vi "CommandFIFOMultiplexer.vi"   [LabVIEW 2018]
uses:
  <vilib>/rvi/Emulation/niFpgaGetClockAttributes.vi
  <vilib>/rvi/Emulation/niFpgaSctlEmulationGetInTimedLoop.vi
  <vilib>/rvi/Emulation/niFpgaEmulationReportErrorSimple.vi
  <vilib>/rvi/interface/RandomDataEmulation/niFpgaRandomDataHandleErrors.vi
  <vilib>/rvi/Emulation/niFpgaEmulationIsFPGAContextNoSignature.vi
  <vilib>/rvi/errors/niFpgaSetErrorForExecOnDevCompSimple.vi
  <vilib>/rvi/eio/common/nirviEmuReportErrorAndStop.vi
  <vilib>/rvi/DataTransferAndStorage/Container/Common/niFpgaContainerGetUniqueNameForEmu.vi
  <vilib>/rvi/FIFO/Fifo_Resource/nirvififoEmulationSetSize.vi
  <vilib>/rvi/FIFO/Fifo_Resource/nirviFifoEmulationQueueMgr.vi
  <instcachedir>/0/nirviFifoEmulationQueueMgr_E5CAEC123FF24DC58D834DCA3CDAA9B5.lvgen/nirviFifoEmulationQueueMgr_E5CAEC123FF24DC58D834DCA3CDAA9B5_001.vi
  <vilib>/rvi/FIFO/Fifo_Resource/nirvififoEmulationDetermineInputValidOut.vi
  <vilib>/rvi/FIFO/Fifo_Resource/nirvififoEmulationCreateLock.vi
  <vilib>/rvi/Emulation/niFpgaProcessEmulError.vi
  <vilib>/rvi/FIFO/Fifo_Resource/nirvififoEmulationObtainLock.vi
  <vilib>/rvi/FIFO/Fifo_Resource/nirvififoEmulationReleaseLock.vi
  <vilib>/rvi/occurrence/nirviWaitOnOccurrenceBase.vi
  <vilib>/rvi/errors/nirviReportUnexpectedCaseInternalError.vi
  <vilib>/rvi/errors/nirviReportUnexpectedCaseInternalError (U32).vi
  <vilib>/rvi/DataTransferAndStorage/Container/Common/niFpgaContainerExecOnDevCompGetState.vi
  <instcachedir>/0/nirviFifoEmulationQueueMgr_E5CAEC123FF24DC58D834DCA3CDAA9B5.lvgen/nirviFifoEmulationQueueMgr_E5CAEC123FF24DC58D834DCA3CDAA9B5_012.vi
  <vilib>/Utility/error.llb/Clear Errors.vi
  <vilib>/rvi/Emulation/niFpgaCriticalErrorInLSC.vi
  <vilib>/rvi/DataTransferAndStorage/Container/XNode/niFpgaContainer.xnode
  <vilib>/rvi/interface/RandomDataEmulation/nirviRandomDataFpgaReadWriteTemplate.vi
  <vilib>/rvi/FIFO/Fifo_Resource/nirvififoEmulationWrite.vi
  <vilib>/rvi/FIFO/Fifo_Resource/niFpgaFifoEmulationRefIn.vi
types:
  T1 = typedef "Addresses.ctl" = enum8{"NA", "Slot1/AI0-CT7Current", "Slot1/AI1-CT8Current", "Slot1/AI2", "Slot1/AI3", "Slot1/AI4", "Slot1/AI5", "Slot1/AI6", "Slot1/AI7", "Slot1/AI8-MixingValvePosition", "Slot1/AI9", "Slot1/AI10", "Slot1/AI11", "Slot1/AI12", "Slot1/AI13", "Slot1/AI14", "Slot1/AI15", "Slot2/AO0-MixingValvePosition", "Slot2/AO1", "Slot2/AO2", "Slot2/AO3", "Slot3/DIO0-ModbusARx", "Slot3/DIO1", "Slot3/DIO2", "Slot3/DIO3", "Slot3/DIO4-ModbusATx", "Slot3/DIO5", "Slot3/DIO6", "Slot3/DIO7", "Slot4/DI0-PS14Status", "Slot4/DI1-PS15Status", "Slot4/DI2-PS16Status", "Slot4/DI3-CtrlRedundancyStatus", "Slot4/DI4-FanCoilDiffuserStatus", "Slot4/DI5-ACPowerCB15Status", "Slot4/DI6-UtilityOutletCB18Status", "Slot4/DI7-CoolandPumpOLStatus", "Slot4/DI8", "Slot4/DI9", "Slot4/DI10", "Slot4/DI11", "Slot4/DI12", "Slot4/DI13", "Slot4/DI14", "Slot4/DI15", "Slot4/DI16-FCHeatersOffInterlock", "Slot4/DI17-CoolandPumpOffInterlock", "Slot4/DI18-GISHBLostInterlock", "Slot4/DI19-MixingValveClosedInterlock", "Slot4/DI20-SupportSystemHBLostInterlock", "Slot4/DI21-CellDoorOpenInterlock", "Slot4/DI22-GISEarthQuakeInterlock", "Slot4/DI23-CoolantPumpEStopInterlock", "Slot4/DI24-CabinetOverTempInterlock", "Slot4/DI25", "Slot4/DI26", "Slot4/DI27", "Slot4/DI28", "Slot4/DI29", "Slot4/DI30", "Slot4/DI31", "Slot5/Ch0-FanCoilHeatersOn", "Slot5/Ch1-ThermalHeartbeat", "Slot5/Ch2-CoolantPumpOn", "Slot5/Ch3", "Slot5/Ch4", "Slot5/Ch5", "Slot5/Ch6", "Slot5/Ch7", "Slot6/Port1-VFD", "Slot6/Port2-FlowMeter", "Slot6/Port3-WindSensor", "Slot6/Port4", "Slot7/Port1", "Slot7/Port2", "Slot7/Port3", "Slot7/Port4", "Slot8/TC0-AirMirrorTopSurface", "Slot8/TC1-MirrorCellAir", "Slot8/TC2-MirrorCoolantSupply", "Slot8/TC3-MirrorCoolandReturn", "Slot8/TC4-TelescopeCoolantSupply", "Slot8/TC5-TelescopeCoolantReturn", "Slot8/TC6", "Slot8/TC7", "Slot8/TC8", "Slot8/TC9", "Slot8/TC10", "Slot8/TC11", "Slot8/TC12", "Slot8/TC13", "Slot8/TC14", "Slot8/TC15", "Undefined17", "Undefined18", "Undefined19", "Undefined20", "Undefined21", "Undefined22", "Undefined23", "Undefined24", "Undefined25", "Undefined26", "Undefined27", "Undefined28", "Undefined29", "Undefined30", "Undefined31", "Undefined32", "Undefined33", "Undefined34", "Undefined35", "Undefined36", "Undefined37", "Undefined38", "Undefined39", "Undefined40", "Undefined41", "Undefined42", "Undefined43", "Undefined44", "Undefined45", "Undefined46", "Undefined47", "Undefined48", "Undefined49", "Undefined50", "Undefined51", "Undefined52", "Undefined53", "Undefined54", "Undefined55", "Undefined56", "Undefined57", "Undefined58", "Undefined59", "Undefined60", "Undefined61", "Undefined62", "Undefined63", "Undefined64", "Undefined65", "Undefined66", "Undefined67", "Undefined68", "Undefined69", "Undefined70", "Undefined71", "Undefined72", "Undefined73", "Undefined74", "Undefined75", "Undefined76", "Undefined77", "Undefined78", "Undefined79", "Undefined80", "Undefined81", "Undefined82", "Undefined83", "Undefined84", "Undefined85", "Undefined86", "Undefined87", "Undefined88", "Undefined89", "Undefined90", "Undefined91", "Undefined92", "Undefined93", "Undefined94", "Undefined95", "Undefined96", "Undefined97", "Undefined98", "Undefined99", "Undefined100", "Undefined101", "Undefined102", "Undefined103", "Undefined104", "Undefined105", "Undefined106", "Undefined107", "Undefined108", "Undefined109", "Undefined110", "Undefined111", "Undefined112", "Undefined113", "Undefined114", "Undefined115", "Undefined116", "Undefined117", "Undefined118", "Undefined119", "Undefined120", "Undefined121", "Undefined122", "Undefined123", "Undefined124", "Undefined125", "Undefined126", "Undefined127", "Undefined128", "Undefined129", "Undefined130", "Undefined131", "Undefined132", "Undefined133", "Undefined134", "Undefined135", "Undefined136", "Undefined137", "Undefined138", "Undefined139", "Undefined140", "Undefined141", "Undefined142", "Undefined143", "Undefined144", "Undefined145", "Undefined146", "Undefined147", "Undefined148", "Undefined149", "Undefined150", "Undefined151", "Undefined152", "Undefined153", "Undefined154", "Undefined155", "Undefined156", "Undefined157", "Undefined158", "Undefined159", "Undefined160", "Undefined161", "Undefined162", "Undefined163", "Undefined164", "Undefined165", "Undefined166", "Undefined167", "Undefined168", "Undefined169", "Undefined170", "Undefined171", "Undefined172", "Undefined173", "Undefined174", "Undefined175", "ModbusSoftwareTrigger", "Telemetry", "HealthAndStatus", "Timestamp"}
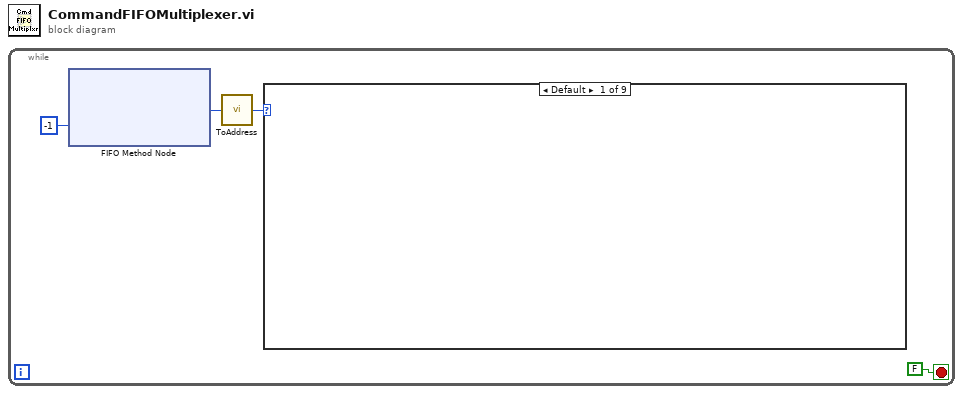
[diagram p0: block diagram]
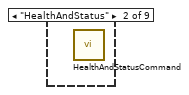
[diagram p2: hidden frame]
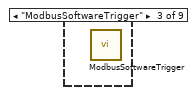
[diagram p3: hidden frame]
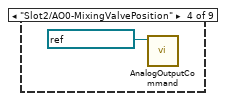
[diagram p4: hidden frame]
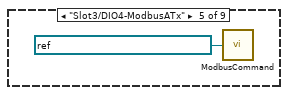
[diagram p5: hidden frame]
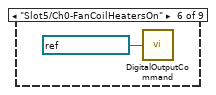
[diagram p6: hidden frame]
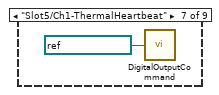
[diagram p7: hidden frame]
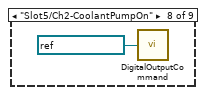
[diagram p8: hidden frame]
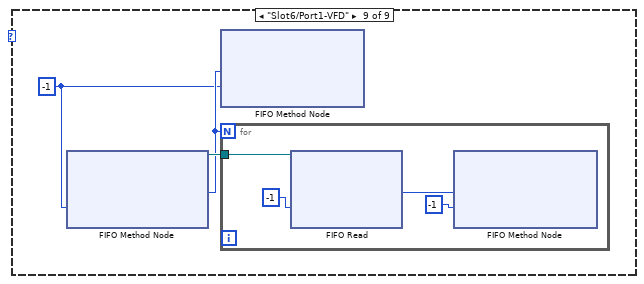
[diagram p9: hidden frame]
diagram:
  n1 = while {
    stop <- FALSE stop-if-true
    n2 = xnode ("FIFO Method Node")("Timeout"=-1) -> ("Element"=w3:u16)  [unwired: 1 in, 2 out]
    n3 = call "ToAddress.vi"("Input"=w3) -> ("Address"=w2:T1)
    n4 = case shown="Default" w2 {
      frame Default {
      }
      frame "HealthAndStatus" {
        n5 = call "HealthAndStatusCommand.vi"() -> ()  [unwired: 12 in]
      }
      frame "ModbusSoftwareTrigger" {
        n6 = call "ModbusSoftwareTrigger.vi"() -> ()  [unwired: 12 in]
      }
      frame "Slot2/AO0-MixingValvePosition" {
        n7 = call "AnalogOutputCommand.vi"("FPGA I/O In"=refnum<k21> "Mod2/AO0") -> ()  [unwired: 11 in]
      }
      frame "Slot3/DIO4-ModbusATx" {
        n8 = call "ModbusCommand.vi"("SubnetTxFIFO"=refnum<k21> "ModbusSubnetATxDataFIFO") -> ()  [unwired: 1 in]
      }
      frame "Slot5/Ch0-FanCoilHeatersOn" {
        n9 = call "DigitalOutputCommand.vi"("FPGA I/O In"=refnum<k21> "Mod5/CH0") -> ()  [unwired: 1 in]
      }
      frame "Slot5/Ch1-ThermalHeartbeat" {
        n10 = call "DigitalOutputCommand.vi"("FPGA I/O In"=refnum<k21> "Mod5/CH1") -> ()  [unwired: 1 in]
      }
      frame "Slot5/Ch2-CoolantPumpOn" {
        n11 = call "DigitalOutputCommand.vi"("FPGA I/O In"=refnum<k21> "Mod5/CH2") -> ()  [unwired: 1 in]
      }
      frame "Slot6/Port1-VFD" {
        w10 = -1 ("Timeout")
        n12 = xnode ("FIFO Method Node")("Timeout"=w10) -> ("Element"=w11:u16, "FIFO Out"=w12:refnum<k21>)  [unwired: 1 in, 1 out]
        n13 = xnode ("FIFO Method Node")("Element"=w11, "Timeout"=w10) -> ()  [unwired: 1 in, 2 out]
        n14 = for {
          N: w11 -> [_]
          tunnel: w12 -> [w16]
          n15 = xnode ("FIFO Read")("Timeout"=-1, "FIFO In"=w16) -> ("Element"=w14:u16)  [unwired: 2 out]
          n16 = xnode ("FIFO Method Node")("Element"=w14, "Timeout"=-1) -> ()  [unwired: 1 in, 2 out]
        }
      }
    }
  }
